vi "Live stim trig width abs lim.vi"(11 "Live stim.trig.width (ms)":dbl) -> (3 "Live stim.trig.width (ms)":dbl)   [LabVIEW 2013]
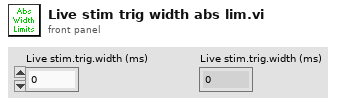
[diagram p1: front panel]
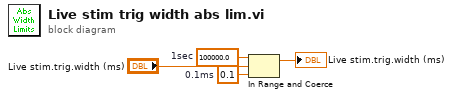
[diagram p0: block diagram]
diagram:
  w2 = 100000.0  # 1sec
  w1 = 0.1  # 0.1ms
  n1 = In Range and Coerce(upper limit=w2, x="Live stim.trig.width (ms)", lower limit=w1) -> (coerced(x)=→"Live stim.trig.width (ms)":dbl)  [unwired: 1 out]
